vi "Write Attributes Metadata.vi"(10 "Attributes Metadata":refnum<class "Attributes Metadata.lvclass">, 11 "Base Attributes in":refnum<class "Base Attributes.lvclass">) -> (3 "Base Attributes out":refnum<class "Base Attributes.lvclass">)   [LabVIEW 2020, in "jettl.lvlib" / "Base Attributes.lvlib" / "Base Attributes.lvclass"]
uses:
  Base Attributes.lvclass
  Attributes Metadata/Attributes Metadata.lvclass
  Base Attributes.lvclass/Base Attributes.ctl
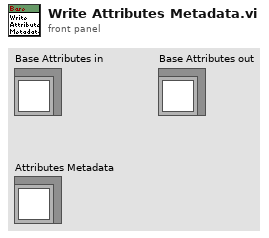
[diagram p1: front panel]
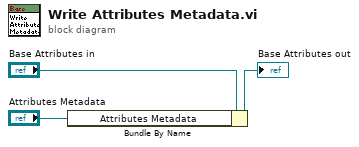
[diagram p0: block diagram]
diagram:
  n1 = Bundle By Name(cluster="Base Attributes in", "Attributes Metadata"="Attributes Metadata") -> (→"Base Attributes out":refnum<class "Base Attributes.lvclass">)
